vi "build_xywav.vi"(1 "x0":dbl, 2 "dx":dbl=1.0, 3 "x units":string="index", 4 "x dim":string="x", 7 "z data":dbl[][](array[numeric])=array100x1024[102400 elements], 9 "z units":string="au", 11 "attributes":variant, 12 "y0":dbl, 13 "dy":dbl=1.0, 14 "y units":string="index", 15 "y dim":string="y") -> (8 "xywave":T1={"attributes"=variant, "Z"={"data"=[], "units"="au"}, "X"={"start"=0.0, "delta"=1.0, "units"="index", "dim"="x"}, "Y"={"start"=0.0, "delta"=1.0, "units"="index", "dim"="y"}})   [LabVIEW 2015]
uses:
  xywav.ctl
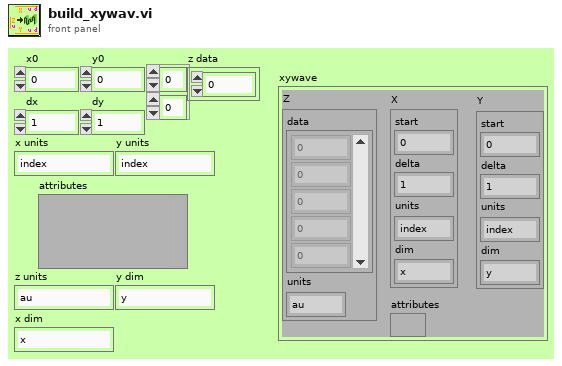
[diagram p1: front panel]
types:
  T1 = typedef "xywav.ctl" = cluster{"attributes":variant, "Z":cluster{"data":dbl[][], "units":string}, "X":cluster{"start":dbl, "delta":dbl, "units":string, "dim":string}, "Y":cluster{"start":dbl, "delta":dbl, "units":string, "dim":string}}
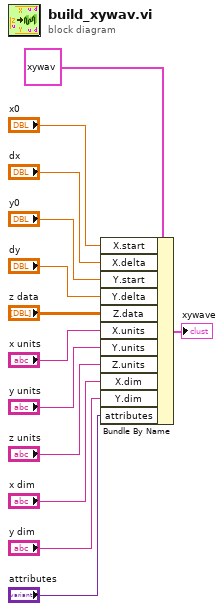
[diagram p0: block diagram]
diagram:
  n1 = Bundle By Name(cluster=T1 {"attributes"=variant, "Z"={"data"=[], "units"="au"}, "X"={"start"=0.0, "delta"=0.0, "units"="index", "dim"="index"}, "Y"={"start"=0.0, "delta"=0.0, "units"="index", "dim"="index"}} ("xywave"), "X.start"="x0", "X.delta"="dx", "Y.start"="y0", "Y.delta"="dy", "Z.data"="z data", "X.units"="x units", "Y.units"="y units", "Z.units"="z units", "X.dim"="x dim", "Y.dim"="y dim", "attributes"="attributes") -> (→"xywave":T1)
